vi "16T_Open_Queue.vi"(8 "error in (no error)":errorcluster) -> (0 "error out":errorcluster, 2 "queue out":refnum<queue>)   [LabVIEW 2016]
uses:
  Gustav/20TVTI_Control.ctl
  Global/Global Variables/Queues_global.vi
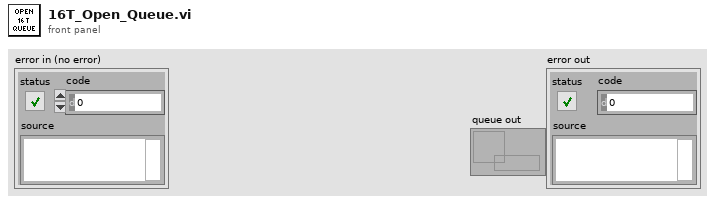
[diagram p1: front panel]
types:
  T1 = typedef "20TVTI_Control.ctl" = cluster{"Set VTI SP":bool, "Change NV Status":bool, "Set NV Setpoint":bool, "Change Heater Status":bool, "Set D-Heater Setpoint":bool, "Set Heater Setpoint":bool, "Change D-Heater Status":bool, "Set Sweep Type":bool, "Setpoint (K)":dbl, "Rate (K/min)":dbl, "Setpoint Heater":dbl, "Setpoint D-Heater":dbl, "Setpoint NV":dbl}
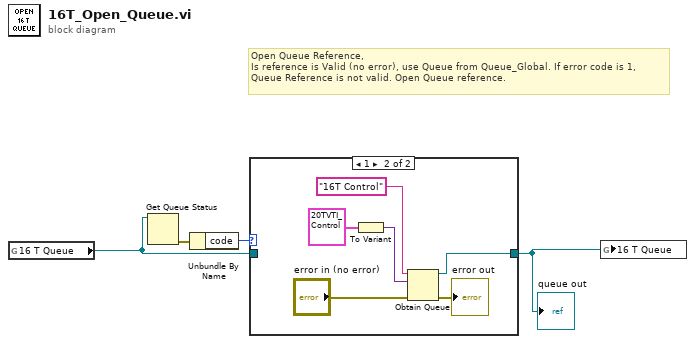
[diagram p0: block diagram]
diagram:
  # "Open Queue Reference, \nIs reference is Valid (no error), use Queue from Queue_Global. If error code is 1, \nQueue Reference is not valid. Open Queue reference."
  n1 = global read "Queues_global.vi" "16 T Queue"() -> (w2:refnum<queue>)
  n2 = Get Queue Status(queue=w2) -> (error out=w4:errorcluster)  [unwired: 2 in, 7 out]
  n3 = Unbundle By Name(w4) -> ("code"=w3:i32)
  n4 = case shown="1" w3 {
    tunnel: [w5 w6] -> w1
    tunnel: w2 -> [w5 _]
    frame 0, Default {
    }
    frame 1 {
      n5 = To Variant(anything=T1 {"Set VTI SP"=FALSE, "Change NV Status"=FALSE, "Set NV Setpoint"=FALSE, "Change Heater Status"=FALSE, "Set D-Heater Setpoint"=FALSE, "Set Heater Setpoint"=FALSE, "Change D-Heater Status"=FALSE, "Set Sweep Type"=FALSE, "Setpoint (K)"=0.0, "Rate (K/min)"=0.0, "Setpoint Heater"=0.0, "Setpoint D-Heater"=0.0, "Setpoint NV"=0.0} ("Cluster")) -> (Variant=w10:variant)
      n6 = Obtain Queue(name (unnamed)="16T Control", element data type=w10, error in (no error)="error in (no error)") -> (queue out=w6:refnum<queue>, error out=→"error out":errorcluster)  [unwired: 2 in, 1 out]
    }
  }
  "queue out" <- w1
  n7 = global write "Queues_global.vi" "16 T Queue"(w1) -> ()
